vi "Test - Connector Pane.vi"() -> ()   [LabVIEW 2019]
doc: "This VI is used in conjunction with the Add Terminals to Connector Pane.vi example. That VI will manipulate this VI's connector pane."
panel:
  in  "String":string
  out "Waveform Graph":dbl[](graph)
  in  "Table":string[][](table)
  in  "Listbox":i32(listbox)
  in  "Menu Ring":u16(ring) items=["test"]
  in  "Boolean":bool
  in  "Numeric":dbl
  # "This VI is used in conjunction with Add Terminals to Connector Pane.vi. That VI will modify this VI's connector pane."
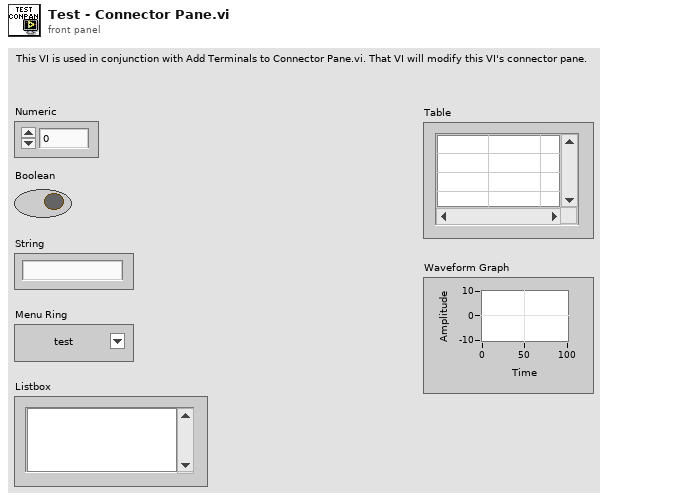
[diagram p1: front panel]
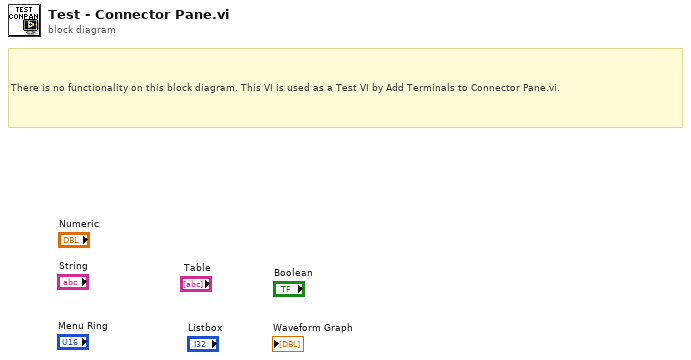
[diagram p0: block diagram]
diagram:
  # "There is no functionality on this block diagram. This VI is used as a Test VI by Add Terminals to Connector Pane.vi."
